vi "Get HW Config.vi"(8 "error in":errorcluster) -> (0 "error out":errorcluster)   [LabVIEW 2019, in "SEECD System Explorer.lvlib"]
uses:
  SEECD System Explorer.lvlib
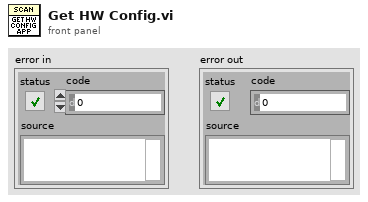
[diagram p1: front panel]
types:
  T1 = typedef "SEECD System Explorer.lvlib/Host - HW Config.ctl" = cluster{"Local Chassis":T2, "Masters":T5[]}
  T2 = typedef "SEECD System Explorer.lvlib/Host - Local Chassis.ctl" = cluster{"Modules":T3[]}
  T3 = typedef "SEECD System Explorer.lvlib/Host - Module.ctl" = cluster{"IOV Ref":string, "Slot":u32, "Model":u32, "All Variables":T4[]}
  T4 = typedef "SEECD System Explorer.lvlib/IOV Container Contents.ctl" = cluster{"Name":string, "Writable":bool, "DataType":variant}
  T5 = typedef "SEECD System Explorer.lvlib/Host - Master.ctl" = cluster{"IOV Ref":string, "Name":string, "Master ID":u32, "Slaves":T6[]}
  T6 = typedef "SEECD System Explorer.lvlib/Host - Slave.ctl" = cluster{"IOV Ref":string, "Name":string, "Position Address":u16, "Bitfile Signature":u8[], "Modules":T3[], "ECAT IOV Contents":T4[]}
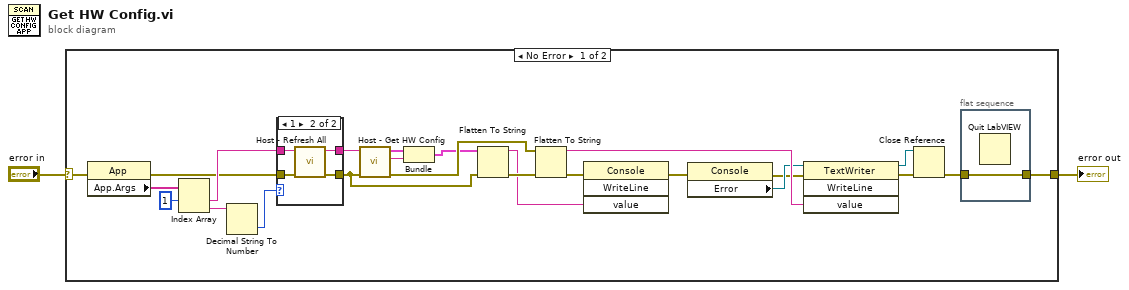
[diagram p0: block diagram]
diagram:
  n1 = case shown="No Error" "error in" {
    selector: "error in" -> [w25 w34]
    tunnel: [w23 w34] -> w2
    frame No Error {
      n2 = property class="App"(error in=w25) -> (error out=w9:errorcluster, "App.Args"=w26:string[])  [unwired: 1 in, 1 out]
      n3 = Index Array(array=w26, index #1=1 ("index")) -> (element #1=w10:string, element #2=w8:string)  [unwired: 1 in]
      n4 = Decimal String To Number(string=w8) -> (number=w7:i32)  [unwired: 2 in, 1 out]
      n5 = case shown="1" w7 {
        tunnel: [w28 w33] -> w12
        tunnel: [w29 w32] -> w11
        tunnel: w10 -> [w29 w31]
        tunnel: w9 -> [w28 w30]
        frame 0, Default {
        }
        frame 1 {
          n6 = call "Host - Refresh All.vi"("error in (no error)"=w30, "serverName"=w31) -> ("error out"=w33:errorcluster, "serverName"=w32:string)  [unwired: 8 in]
        }
      }
      n7 = call "Host - Get HW Config.vi"("error in (no error)"=w12, "serverName"=w11) -> ("error out"=w13:errorcluster, "Message output"=w4:string, "HW Config"=w5:T1)  [unwired: 7 in]
      n8 = Bundle("HW Config"=w5, "Message output"=w4) -> (w3:cluster{"HW Config":T1, "Message output":string})  [unwired: 1 in]
      n9 = Flatten To String(anything=w3, error in (no error)=w12) -> (data string=w20:string, error out=w22:errorcluster)  [unwired: 2 in, 1 out]
      n10 = Flatten To String(anything=w13, error in (no error)=w22) -> (data string=w19:string, error out=w21:errorcluster)  [unwired: 2 in, 1 out]
      n11 = invoke class="Console" method="WriteLine"(error in=w21, "value"=w20) -> (error out=w6:errorcluster)  [unwired: 2 in, 3 out]
      n12 = property class="Console"(error in=w6) -> (error out=w14:errorcluster, "Error"=w18:refnum<k24>)  [unwired: 1 in, 1 out]
      n13 = invoke class="TextWriter" method="WriteLine"(reference=w18, error in=w14, "value"=w19) -> (reference out=w16:refnum<k24>, error out=w17:errorcluster)  [unwired: 1 in, 2 out]
      n14 = Close Reference(reference=w16, error in (no error)=w17) -> (error out=w15:errorcluster)
      n15 = flat-sequence {
        tunnel: w15 -> [w27]
        tunnel: [w27] -> w23
        frame #0 {
          n16 = Quit LabVIEW() -> ()  [unwired: 1 in]
        }
      }
    }
    frame Error {
    }
  }
  "error out" <- w2
